vi "Read Liquid Status.vi"(8 "error in":errorcluster, 11 "3010 in":refnum<class "3010.lvclass">) -> (0 "error out":errorcluster, 2 "Full?":bool, 3 "3010 out":refnum<class "3010.lvclass">)   [LabVIEW 2012, in "3010.lvclass"]
doc: "Determine whether the liquid resevoir has enough."
uses:
  3010.lvclass
  Controls/CmdStruct.ctl
  Controls/Enum Cmd.ctl
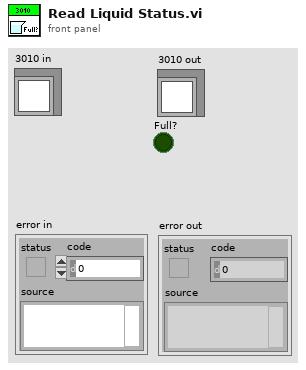
[diagram p1: front panel]
types:
  T1 = typedef "3010.lvclass/Enum Cmd.ctl" = enum16{"Dump", "Dump Cumulative", "Read Liquid Status", "Read Condenser Temperature", "Read Saturator Temperature", "Read Environment", "Read 6 s Buffer", "Read 1 s Buffer", "Read Concentration Display", "Read Delta T", "Read Vacuum Status", "Set Analog Voltage", "Execute Fill", "Clear Display Buffers"}
  T2 = typedef "CmdStruct.ctl" = cluster{"Cmd":u8, "x":i64, "y":i64, "Display":string}
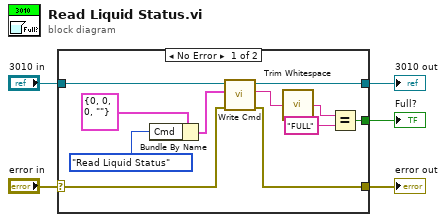
[diagram p0: block diagram]
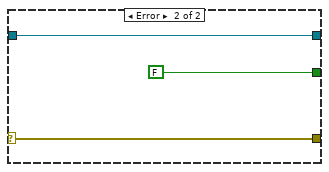
[diagram p2: hidden frame]
diagram:
  n1 = case shown="No Error" "error in" {
    selector: "error in" -> [w14 w19]
    tunnel: [w7 w19] -> w4
    tunnel: [w11 w18] -> w2
    tunnel: "3010 in" -> [w16 w18]
    tunnel: [w6 FALSE] -> w1
    frame No Error {
      n2 = Bundle By Name(cluster=T2 {"Cmd"=0, "x"=0, "y"=0, "Display"=""} ("CmdStruct"), "Cmd"=Enum_Cmd."Read Liquid Status" ("Enum Cmd")) -> (w12:T2)
      n3 = call-dynamic "Write Cmd.vi"("error in"=w14, "CmdStruct"=w12, "CPC in"=w16) -> ("error out"=w7:errorcluster, "Buffer"=w10:string, "CPC out"=w11:refnum<class "3010.lvclass">)  [unwired: 6 in]
      n4 = call <vilib>:"Trim Whitespace.vi"("string"=w10) -> ("trimmed string"=w9:string)  [unwired: 1 in]
      n5 = Equal?(x=w9, y="FULL") -> (x = y?=w6:bool)
    }
    frame Error {
    }
  }
  "error out" <- w4
  "3010 out" <- w2
  "Full?" <- w1
